vi "Machine Cal Data Engine (global).vi"(2 "Mode":T1(ring)=enum."Engine Idle", 7 "Data In":dbl[](array[numeric])) -> (4 "Stream Data":bool, 8 "Data Out":dbl[](array[numeric]), 10 "New Data":bool, 15 "Connection":bool)   [LabVIEW 2013]
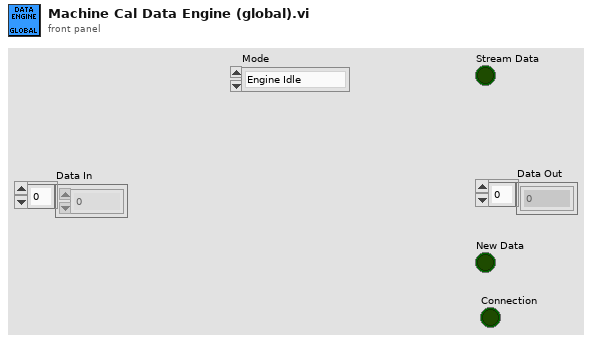
[diagram p1: front panel]
types:
  T1 = enum16{"Init", "Start Data", "Stop Data", "Lost Connection", "Engine Idle", "Write Data", "Read Data"}
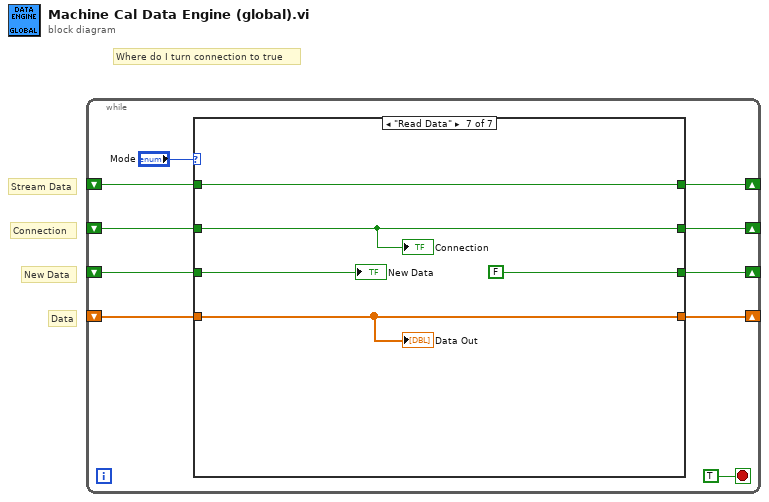
[diagram p0: block diagram]
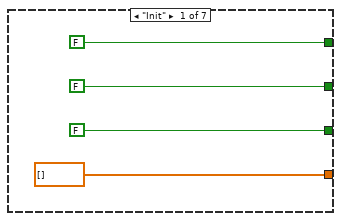
[diagram p2: hidden frame]
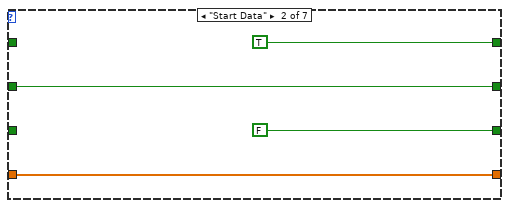
[diagram p3: hidden frame]
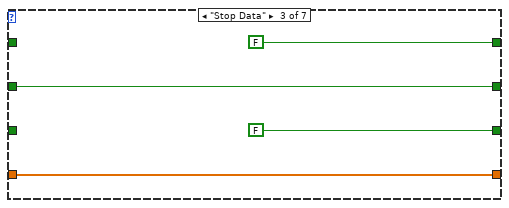
[diagram p4: hidden frame]
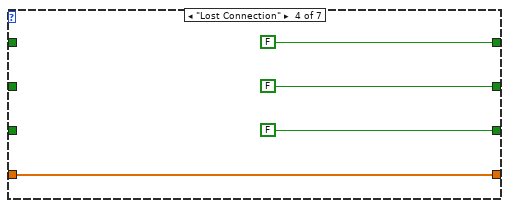
[diagram p5: hidden frame]
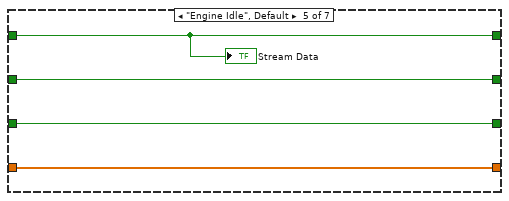
[diagram p6: hidden frame]
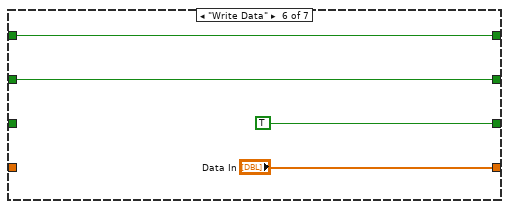
[diagram p7: hidden frame]
diagram:
  # "Data"
  # "New Data"
  # "Connection"
  # "Where do I turn connection to true"
  # "Stream Data"
  n1 = while {
    shift-right: [w8] -> _
    shift-left: _ -> [w7]
    shift-right: [w6] -> _
    shift-left: _ -> [w5]
    shift-right: [w4] -> _
    shift-left: _ -> [w3]
    shift-right: [w2] -> _
    shift-left: _ -> [w1]
    stop <- TRUE stop-if-true
    n2 = case shown="\"Read Data\"" "Mode" {
      tunnel: [FALSE TRUE FALSE FALSE w30 w34 w38] -> w8
      tunnel: w7 -> [_ _ _ _ w30 w34 w38]
      tunnel: [FALSE w17 w21 FALSE w29 w33 w35] -> w6
      tunnel: w5 -> [_ w17 w21 _ w29 w33 w35]
      tunnel: [FALSE FALSE FALSE FALSE w28 TRUE FALSE] -> w4
      tunnel: w3 -> [_ _ _ _ w28 _ w39]
      tunnel: [dbl[] [] w15 w19 w23 w27 "Data In" w36] -> w2
      tunnel: w1 -> [_ w15 w19 w23 w27 _ w36]
      frame "Init" {
      }
      frame "Start Data" {
      }
      frame "Stop Data" {
      }
      frame "Lost Connection" {
      }
      frame "Engine Idle", Default {
        "Stream Data" <- w30
      }
      frame "Write Data" {
      }
      frame "Read Data" {
        "New Data" <- w39
        "Data Out" <- w36
        "Connection" <- w35
      }
    }
  }
